vi "Write Now.vi"(8 "error in (no error)":errorcluster, 10 "Now":dbl, 11 "ExperimentService in":refnum<class "ExperimentService.lvclass">) -> (0 "error out":errorcluster, 3 "ExperimentService out":refnum<class "ExperimentService.lvclass">)   [LabVIEW 2014, in "ExperimentService.lvclass"]
uses:
  ExperimentService.lvclass
  ExperimentService.lvclass/ExperimentService.ctl
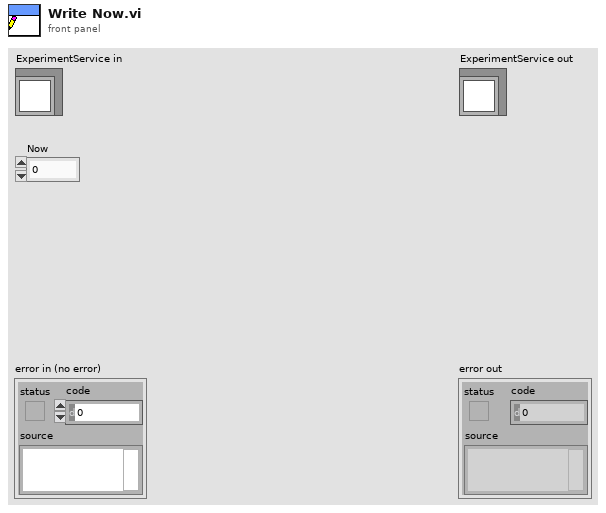
[diagram p1: front panel]
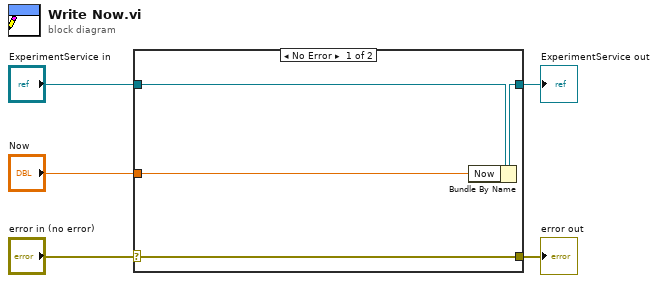
[diagram p0: block diagram]
diagram:
  n1 = case shown="No Error" "error in (no error)" {
    selector: "error in (no error)" -> [w9 w10]
    tunnel: [w9 w10] -> w4
    tunnel: [w7 w11] -> w2
    tunnel: "ExperimentService in" -> [w8 w11]
    tunnel: "Now" -> [w6 _]
    frame No Error {
      n2 = Bundle By Name(cluster=w8, "Now"=w6) -> (w7:refnum<class "ExperimentService.lvclass">)
    }
    frame Error {
    }
  }
  "error out" <- w4
  "ExperimentService out" <- w2
